vi "USBOpen.vi"(8 "error in (no error)":errorcluster, 11 "USB":string="USB0::0x1043::0x0000::NI-VISA-0::RAW") -> (0 "error out":errorcluster, 3 "VISA Resource Name":refnum<visa-resource-name>)   [LabVIEW 2011]
doc: "The vi are opening the specified USB connection."
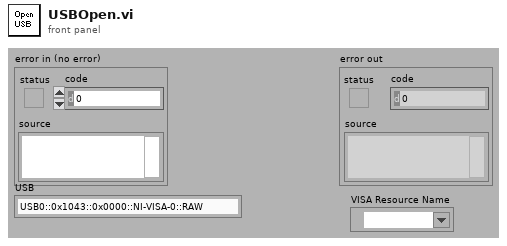
[diagram p1: front panel]
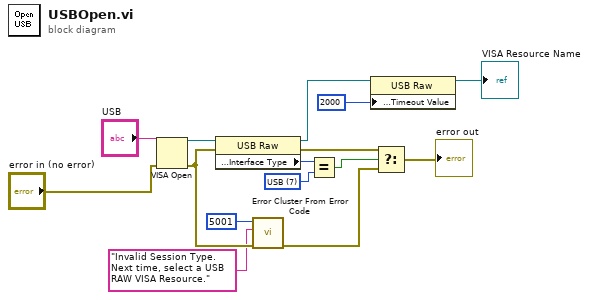
[diagram p0: block diagram]
diagram:
  w12 = u16 7 items=["GPIB"=1, "VXI"=2, "GPIB-VXI"=3, "Serial"=4, "PXI"=5, "TCPIP"=6, "USB"=7] ("Interface Information:Interface Type")
  n1 = VISA Open(error in (no error)="error in (no error)", VISA resource name="USB") -> (VISA resource name=w15:refnum<visa-resource-name>, error out=w10:errorcluster)  [unwired: 3 in]
  n2 = property class="USB Raw"(reference=w15, error in=w10) -> (reference out=w3:refnum<visa-resource-name>, error out=w14:errorcluster, "Interface Information:Interface Type"=w13:u16)
  n3 = call <vilib>:"Error Cluster From Error Code.vi"("error in (no error)"=w10, "error message (\"\")"="Invalid Session Type.  Next time, select a USB RAW VISA Resource." ("error message (\"\")"), "error code (0)"=5001) -> ("error out"=w7:errorcluster)  [unwired: 6 in]
  n4 = Equal?(x=w13, y=w12) -> (x = y?=w11:bool)
  n5 = property class="USB Raw"(reference=w3, "General Settings:Timeout Value"=u32 2000) -> (reference out=→"VISA Resource Name":refnum<visa-resource-name>)  [unwired: 1 in, 1 out]
  n6 = Select(t=w14, s=w11, f=w7) -> (s? t:f=→"error out":errorcluster)
